vi "BuildMsg.vi"(8 "ErrorIn":errorcluster, 9 "AllMessages":bool=TRUE, 10 "AllSender":bool=TRUE, 11 "Result":T2) -> (0 "ErrorOut":errorcluster, 2 "Messages":T3[](array[typedef]))   [LabVIEW 2015]
uses:
  Telegram/Methods/TypeDefs/Message.ctl
  Telegram/Methods/TypeDefs/UpdateUniversal.ctl
  Telegram/Methods/TypeDefs/CommandList.ctl
panel:
  in  "CommandList":T1=["Default", "/getweather", "/led1", "/led2", "/led3", "/gettime", "on", "off", "delete keyboard", "/start"]
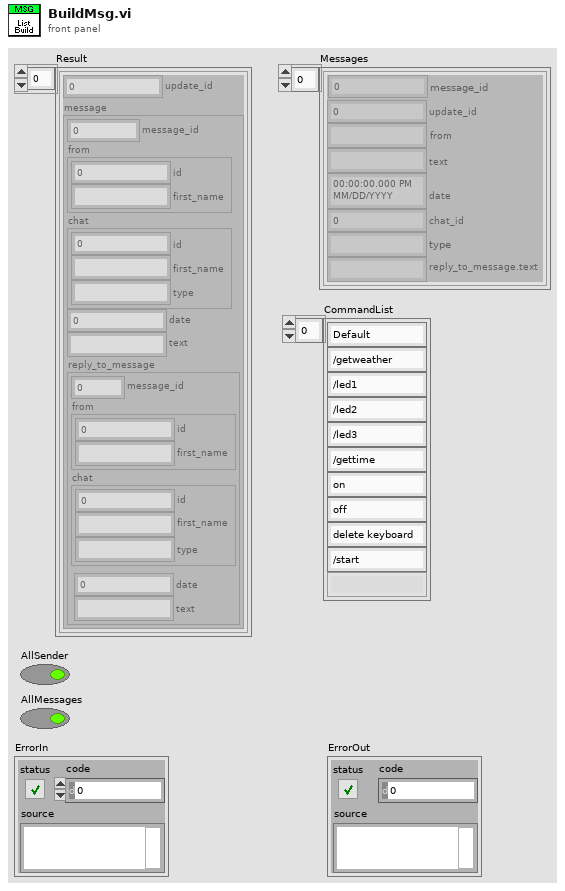
[diagram p1: front panel]
types:
  T1 = typedef "CommandList.ctl" = string[]
  T2 = typedef "UpdateUniversal.ctl" = cluster{"update_id":u32, "message":cluster{"message_id":u32, "from":cluster{"id":u32, "first_name":string}, "chat":cluster{"id":i32, "first_name":string, "type":string}, "date":u32, "text":string, "reply_to_message":cluster{"message_id":u32, "from":cluster{"id":u32, "first_name":string}, "chat":cluster{"id":i32, "first_name":string, "type":string}, "date":u32, "text":string}}}[]
  T3 = typedef "Message.ctl" = cluster{"update_id":u32, "from":string, "text":string, "date":timestamp, "chat_id":i32, "type":string, "reply_to_message.text":string, "message_id":u32}
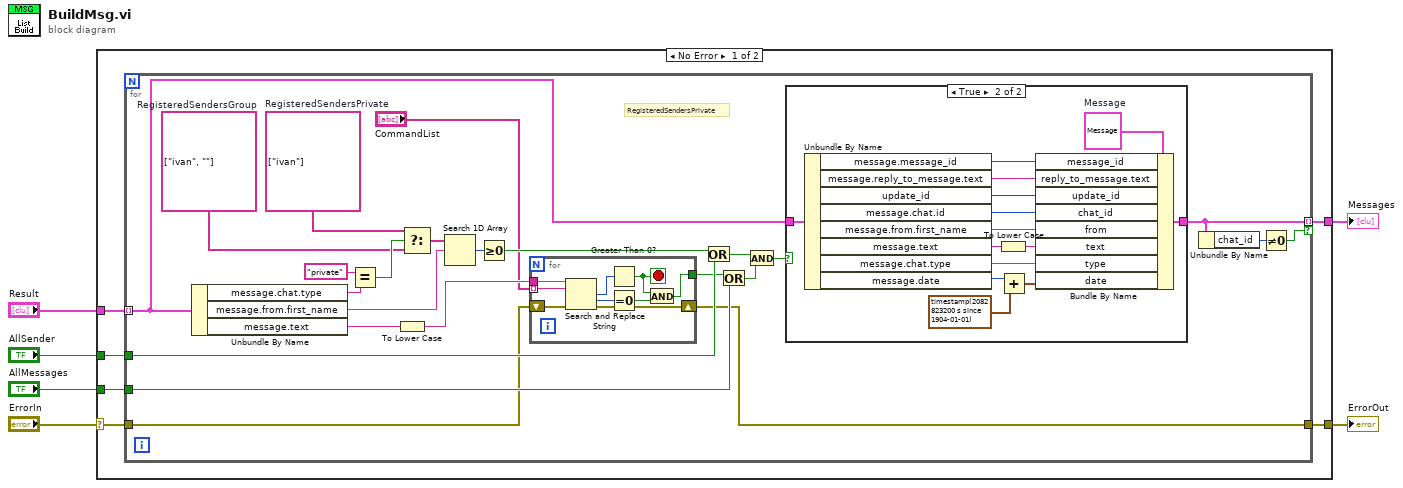
[diagram p0: block diagram]
diagram:
  n1 = case shown="No Error" "ErrorIn" {
    selector: "ErrorIn" -> [w8 w60]
    tunnel: "AllSender" -> [w12 _]
    tunnel: "Result" -> [w11 _]
    tunnel: "AllMessages" -> [w10 _]
    tunnel: [w9 _] -> w2
    tunnel: [w7 w60] -> w3
    frame No Error {
      n2 = for {
        tunnel: w11 -> [w31] mode=indexing
        tunnel: w12 -> [w33]
        tunnel: w10 -> [w18]
        tunnel: [w21] -> w9 mode=indexing if=w19
        tunnel: w8 -> [w16]
        tunnel: [w17] -> w7
        w28 = string[] ["ivan"]  # RegisteredSendersPrivate
        w27 = string[] ["ivan", ""]  # RegisteredSendersGroup
        # "RegisteredSendersPrivate"
        n3 = Unbundle By Name(w31) -> ("message.chat.type"=w26:string, "message.from.first_name"=w35:string, "message.text"=w15:string)
        n4 = Equal?(x="private", y=w26) -> (x = y?=w29:bool)
        n5 = To Lower Case(string=w15) -> (all lower case string=w14:string)
        n6 = Select(t=w28, s=w29, f=w27) -> (s? t:f=w24:string[])
        n7 = Search 1D Array(1D array=w24, element=w35) -> (index of element=w36:i32)  [unwired: 1 in]
        n8 = Greater Or Equal To 0?(x=w36) -> (x >= 0?=w34:bool)
        n9 = for {
          tunnel: "CommandList" -> [w59] mode=indexing
          tunnel: [w54] -> w30
          tunnel: w14 -> [w57]
          shift-right: [w52] -> w17
          shift-left: w16 -> [w51]
          stop <- w53 stop-if-true
          n10 = Search and Replace String(input string=w57, search string=w59, error in=w51) -> (number of replacements=w58:i32, offset past replacement=w56:i32, error out=w52:errorcluster)  [unwired: 5 in, 1 out]
          n11 = Greater Than 0?(x=w58) -> (x > 0?=w53:bool)
          n12 = Equal To 0?(x=w56) -> (x = 0?=w55:bool)
          n13 = And(x=w53, y=w55) -> (x .and. y?=w54:bool)
        }
        n14 = Or(x=w34, y=w33) -> (x .or. y?=w23:bool)
        n15 = Or(x=w30, y=w18) -> (x .or. y?=w22:bool)
        n16 = And(x=w23, y=w22) -> (x .and. y?=w32:bool)
        n17 = case shown="True" w32 {
          tunnel: w31 -> [_ w43]
          tunnel: [_ w39] -> w21
          frame False {
          }
          frame True {
            w49 = T3 {"update_id"=0, "from"="", "text"="", "date"=timestamp(0 s since 1904-01-01), "chat_id"=0, "type"="", "reply_to_message.text"="", "message_id"=0}  # Message
            n18 = Unbundle By Name(w43) -> ("message.message_id"=w40:u32, "message.reply_to_message.text"=w42:string, "update_id"=w44:u32, "message.chat.id"=w48:i32, "message.from.first_name"=w45:string, "message.text"=w38:string, "message.chat.type"=w50:string, "message.date"=w46:u32)
            n19 = To Lower Case(string=w38) -> (all lower case string=w37:string)
            n20 = Add(x=w46, y=timestamp(2082823200 s since 1904-01-01)) -> (x+y=w47:timestamp)
            n21 = Bundle By Name(cluster=w49, "message_id"=w40, "reply_to_message.text"=w42, "update_id"=w44, "chat_id"=w48, "from"=w45, "text"=w37, "type"=w50, "date"=w47) -> (w39:T3)
          }
        }
        n22 = Unbundle By Name(w21) -> ("chat_id"=w20:i32)
        n23 = Not Equal To 0?(x=w20) -> (x != 0?=w19:bool)
      }
    }
    frame Error {
    }
  }
  "ErrorOut" <- w3
  "Messages" <- w2
